vi "相机2影像dtXY-转换成机械手mm.vi"(11 "相机2影像偏移量":T1 {"X" format="%#.3f"}) -> (2 "机械手移动量 mm":T1 {"X" format="%#.3f"})   [LabVIEW 2014]
uses:
  Global.vi
  Controls/XYPos.ctl
panel:
  out "机械手移动量 mm 2":T1 {"X" format="%#.3f"}
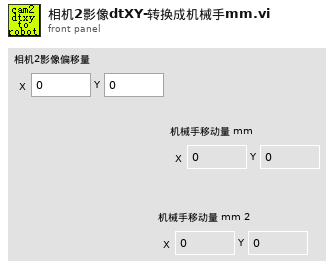
[diagram p1: front panel]
types:
  T1 = typedef "XYPos.ctl" = cluster{"X":dbl, "Y":dbl}
  T2 = typedef "OtherSpec.ctl" = cluster{"其它勾选类规格":T3, "其它数据类规格":T4, "相机名称":T5}
  T3 = typedef "其它勾选类规格.ctl" = cluster{"保存NG图片":bool, "保存OK图片":bool, "保存数据":bool, "开机默认开启监控摄像头":bool}
  T4 = typedef "其他数据类规格.ctl" = cluster{"相机1像素-毫米换算系数":dbl, "相机2像素-毫米换算系数":dbl, "D盘剩余空间预警(G)":dbl, "视频最长录制时间(秒)":dbl}
  T5 = typedef "相机名称品牌使用状态.ctl" = cluster{"相机1名称":T6, "相机2名称":T6, "Cam1启用":bool, "Cam2启用":bool, "Basler1":bool, "Basler2":bool}
  T6 = typedef "IMAQdx.ctl" = refnum<k21>
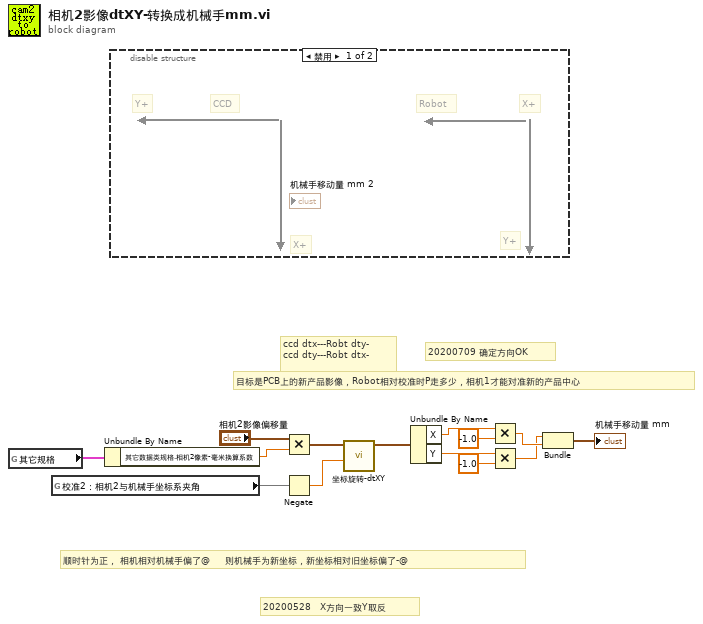
[diagram p0: block diagram]
diagram:
  # "20200709 确定方向OK"
  # "20200528   X方向一致Y取反"
  # "目标是PCB上的新产品影像，Robot相对校准时P走多少，相机1才能对准新的产品中心"
  # "顺时针为正， 相机相对机械手偏了@     则机械手为新坐标，新坐标相对旧坐标偏了-@"
  # "ccd dtx---Robt dty-\nccd dty---Robt dtx-"
  n1 = global read "Global.vi" "其它规格"() -> (w13:T2)
  n2 = global read "Global.vi" "校准2：相机2与机械手坐标系夹角"() -> (w4)
  n3 = Unbundle By Name(w13) -> ("其它数据类规格.相机2像素-毫米换算系数"=w11:dbl)
  n4 = disable-structure shown="禁用" {
    frame Disabled {
      # "CCD"
      # "Y+"
      # "X+"
      # "Y+"
      # "X+"
      # "Robot"
    }
    frame Enabled {
    }
  }
  n5 = Multiply(x="相机2影像偏移量", y=w11) -> (x*y=w14:T1)
  n6 = Negate(x=w4) -> (-x=w3:dbl)
  n7 = call "坐标旋转-dtXY.vi"("旋转角度(单位角度)"=w3, "dtx,dty In"=w14) -> ("dtx,dty Out"=w10:T1)  [unwired: 9 in]
  n8 = Unbundle By Name(w10) -> ("X"=w9:dbl, "Y"=w8:dbl)
  n9 = Multiply(x=w9, y=-1.0) -> (x*y=w2:dbl)
  n10 = Multiply(x=w8, y=-1.0) -> (x*y=w1:dbl)
  n11 = Bundle(w1, w2) -> (→"机械手移动量 mm":cluster{dbl, dbl})  [unwired: 1 in]
